vi "Get Row as String Array.vi"(8 "error in (no error)":errorcluster, 9 "Replace FKs? (F)":bool, 10 "Keep DB Column Order (F)":bool, 11 "Table in":refnum<class "Basic Table.lvclass">) -> (0 "error out":errorcluster, 1 "Row Values":string[](array[string]), 2 "Column Names":string[](array[string]), 3 "Table out":refnum<class "Basic Table.lvclass">)   [LabVIEW 2020, in "Table.lvlib" / "Basic Table.lvclass"]
uses:
  Basic Table.lvclass
  Basic Table.lvclass/Basic Table.ctl
  Column Libraries/Column Interface/Column Interface Class/Column Interface.lvclass
  Table Configuration Interface/Table Configuration Interface.lvclass
  Database Libraries/Database Interfaces/Database Interface Class/Database Interface.lvclass
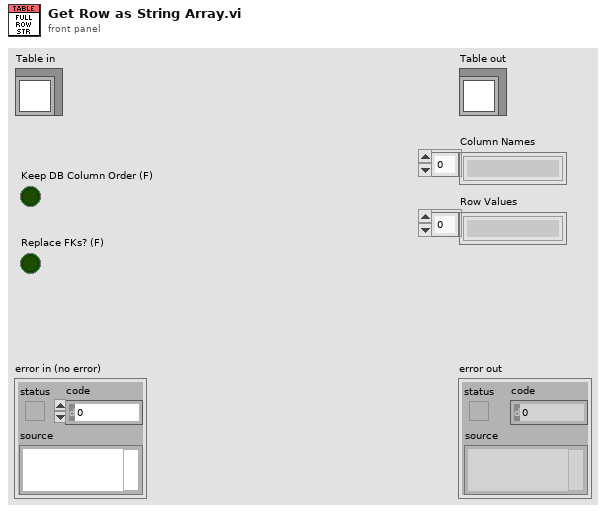
[diagram p1: front panel]
types:
  T1 = map{string, refnum<class "Column Interface.lvclass">}
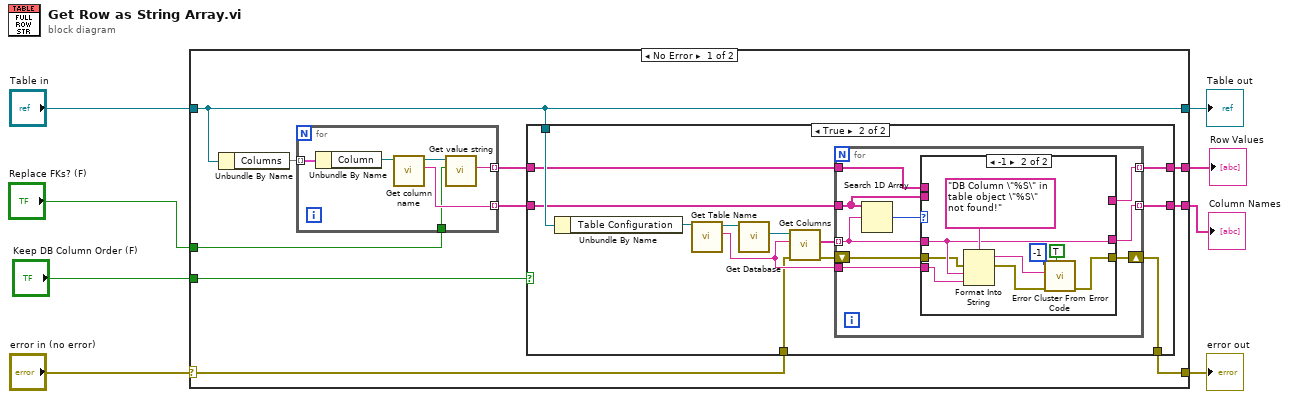
[diagram p0: block diagram]
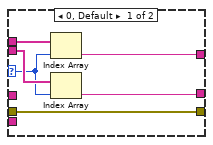
[diagram p3: hidden frame]
diagram:
  n1 = case shown="No Error" "error in (no error)" {
    selector: "error in (no error)" -> [w10 w66]
    tunnel: [w11 w66] -> w7
    tunnel: [w12 w65] -> w5
    tunnel: "Table in" -> [w12 w65]
    tunnel: [w13 _] -> w4
    tunnel: [w14 _] -> w3
    tunnel: "Keep DB Column Order (F)" -> [w17 _]
    tunnel: "Replace FKs? (F)" -> [w9 _]
    frame No Error {
      n2 = Unbundle By Name(w12) -> ("Columns"=w18:T1)
      n3 = for {
        tunnel: w18 -> [w63] mode=indexing
        tunnel: [w61] -> w15 mode=indexing
        tunnel: [w60] -> w16 mode=indexing
        tunnel: w9 -> [w59]
        n4 = Unbundle By Name(w63) -> ("Column"=w62:refnum<class "Column Interface.lvclass">)
        n5 = call-dynamic "Get column name.vi"("Column Interface in"=w62) -> ("Name"=w61:string, "Column Interface out"=w64:refnum<class "Column Interface.lvclass">)  [unwired: 8 in, 1 out]
        n6 = call-dynamic "Get value string.vi"("Replace FKs? (F)"=w59, "Column Interface in"=w64) -> ("Value"=w60:string)  [unwired: 7 in, 2 out]
      }
      n7 = case shown="True" w17 {
        tunnel: w16 -> [w21 w28]
        tunnel: w15 -> [w20 w29]
        tunnel: [w21 w27] -> w14
        tunnel: [w20 w26] -> w13
        tunnel: w12 -> [_ w34]
        tunnel: [w19 w23] -> w11
        tunnel: w10 -> [w19 w22]
        frame False {
        }
        frame True {
          n8 = Unbundle By Name(w34) -> ("Table Configuration"=w33:refnum<class "Table Configuration Interface.lvclass">)
          n9 = call-dynamic "Get Table Name.vi"("Table Configuration Interface in"=w33) -> ("Table Name"=w25:string, "Table Configuration Interface out"=w32:refnum<class "Table Configuration Interface.lvclass">)  [unwired: 8 in, 1 out]
          n10 = call-dynamic "Get Database.vi"("Table Configuration Interface in"=w32) -> ("Database"=w31:refnum<class "Database Interface.lvclass">)  [unwired: 8 in, 2 out]
          n11 = call-dynamic "Get Columns.vi"("error in (no error)"=w22, "Table Name"=w25, "Database Interface in"=w31) -> ("error out"=w24:errorcluster, "Column Name Array"=w30:string[])  [unwired: 6 in, 1 out]
          n12 = for {
            tunnel: w30 -> [w38] mode=indexing
            tunnel: w29 -> [w41]
            tunnel: w28 -> [w42]
            tunnel: [w40] -> w27 mode=indexing
            tunnel: [w39] -> w26 mode=indexing
            tunnel: w25 -> [w37]
            shift-right: [w35] -> w23
            shift-left: w24 -> [w36]
            n13 = Search 1D Array(1D array=w41, element=w38) -> (index of element=w43:i32)  [unwired: 1 in]
            n14 = case shown="-1" w43 {
              selector: w43 -> [w47 _]
              tunnel: w42 -> [w49 _]
              tunnel: w41 -> [w48 _]
              tunnel: [w46 _] -> w40
              tunnel: [w45 w57] -> w39
              tunnel: w38 -> [_ w57]
              tunnel: w37 -> [_ w56]
              tunnel: w36 -> [w44 w53]
              tunnel: [w44 w50] -> w35
              frame 0, Default {
                n15 = Index Array(array=w49, index=w47) -> (element=w46:string)
                n16 = Index Array(array=w48, index=w47) -> (element=w45:string)
              }
              frame -1 {
                n17 = Format Into String(format string="DB Column \"%S\" in table object \"%S\" not found!", error in=w53, w57, w56) -> (resulting string=w52:string, error out=w51:errorcluster)  [unwired: 1 in]
                n18 = call <vilib>:"Error Cluster From Error Code.vi"("show call chain? (False)"=TRUE, "error in (no error)"=w51, "error message (\"\")"=w52, "error code (0)"=-1) -> ("error out"=w50:errorcluster)  [unwired: 5 in]
              }
            }
          }
        }
      }
    }
    frame Error {
    }
  }
  "error out" <- w7
  "Table out" <- w5
  "Column Names" <- w4
  "Row Values" <- w3
